vi "Main Remote MSS test.vi"() -> ()   [LabVIEW 2023]
uses:
  <vilib>/ni/Actors/Network Endpoint Actors/Protocols/Network Stream Strategy/Netowrk Stream Listener/Network Stream Listener.lvclass
  MSS/Lock-In Remote Actor/Lock-In Remote Actor.lvclass
  MSS/MSS Remote Actor/MSS Remote Actor.lvclass
panel:
  out "error out":errorcluster
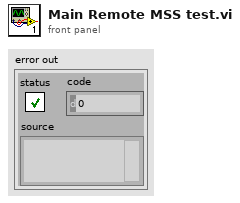
[diagram p1: front panel]
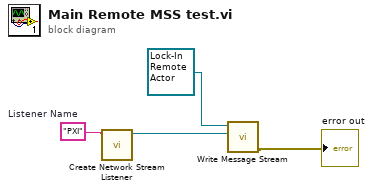
[diagram p0: block diagram]
diagram:
  w3 = "PXI"  # Listener Name
  n1 = call <vilib>:"Create Network Stream Listener.vi"("Name"=w3) -> ("Network Stream Listener"=w4:refnum<class "Network Stream Listener.lvclass">)  [unwired: 10 in]
  n2 = call "Write Message Stream.vi"("Message Stream.lvclass"=w4, "MSS Actor in"=refnum<class "Lock-In Remote Actor.lvclass"> refnum ("Lock-In Remote Actor.lvlib:Lock-In Remote Actor.lvclass")) -> ("error out"=→"error out":errorcluster)  [unwired: 8 in, 1 out]
